vi "XIPIN_Motion_Adaptive_Noise_Reduction_5_01_a.vi"   [LabVIEW 2017]
doc: "The Xilinx Motion Adaptive Noise Reduction LogiCORE is an effective module for both motion detection and motion adaptive noise reduction in video streams. The core allows the motion detection function to be used independently of the noise reduction function for applications where noise reduction is not needed. The noise reduction algorithm is implemented as a recursive temporal filter with a user programmable transfer function allowing the user to control both the shape of the motion transfer and the strength of the noise reduction applied. The user may select either a parameterizable dynamically-configurable AXI4-Lite netlist or a Constant interface netlist. The AXI4-Lite core enables a microprocessor or external state-machine to program MANR parameters and load a Motion Transfer function in real time..\n------------------------------------\n<b>Need License</b> : Yes\n<b>Interface</b> : AXI4-Stream AXI4-Lite"
uses:
  <vilib>/rvi/XilinxIP/XIPIN_XNode/niFpgaXIPIN.xnode
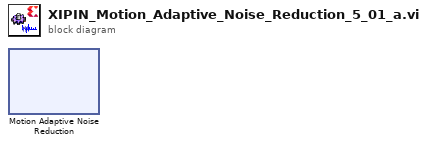
[diagram p0: block diagram]
diagram:
  n1 = xnode ("Motion Adaptive Noise Reduction")() -> ()
